vi "feedforward.vi"(9 "w_times_x":dbl format="%#_13g", 10 "w_times_y":dbl format="%#_13g", 11 "w_times_z":dbl format="%#_13g") -> (0 "Output (0to1)":dbl)   [LabVIEW 2014]
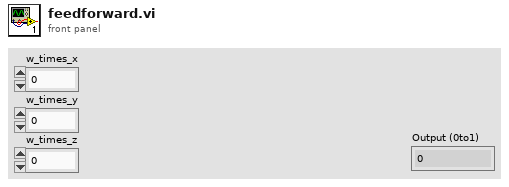
[diagram p1: front panel]
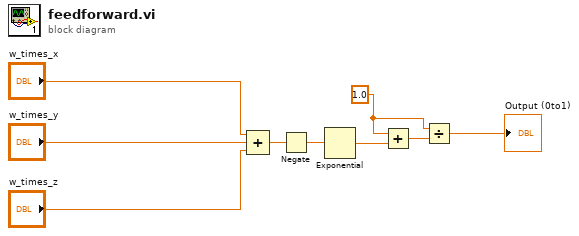
[diagram p0: block diagram]
diagram:
  w8 = 1.0 ("x")
  n1 = Compound Arithmetic op=ADD("w_times_x", "w_times_y", "w_times_z") -> (w6:dbl)
  n2 = Negate(x=w6) -> (-x=w9:dbl)
  n3 = Exponential(1:w9) -> (0:w5:dbl)
  n4 = Add(x=w8, y=w5) -> (x+y=w7:dbl)
  n5 = Divide(x=w8, y=w7) -> (x/y=→"Output (0to1)":dbl)
